vi "ROS_Service_Setup.vi"(4 "Msg to Send":string, 5 "Subscriber":T4, 6 "Log in":path, 7 "ROS":T1={"topic port"=1236, "Node"="/labview", "topic"="/robot/head/command_head_nod", "type"="std_msgs/Bool", "node port"=7000, "error "={"status"=FALSE, "code"=0, "source"=""}, "Direction"=enum."Publisher", "APIs"=[], "Update (ms)"=1, "write queue"=1}, 8 "Log in":T3[](array[typedef])) -> (0 "Log out":path, 1 "Success?":bool, 2 "Reply":string, 3 "Log out":T3[](array[typedef]))   [LabVIEW 2012]
doc: "Creates and sends the connection header and message to a service provider. Implemented in the background server."
uses:
  <userlib>/ROSforLV/ROS/Code/Console/Servers/ServerSubs/ROSLog.ctl
  <userlib>/ROSforLV/ROS/Code/SubVIs/_ROSControl.ctl
  <userlib>/ROSforLV/ROS/Code/SubVIs/_ROSDirection.ctl
  <userlib>/ROSforLV/ROS/Code/_ROSDefinition.vi
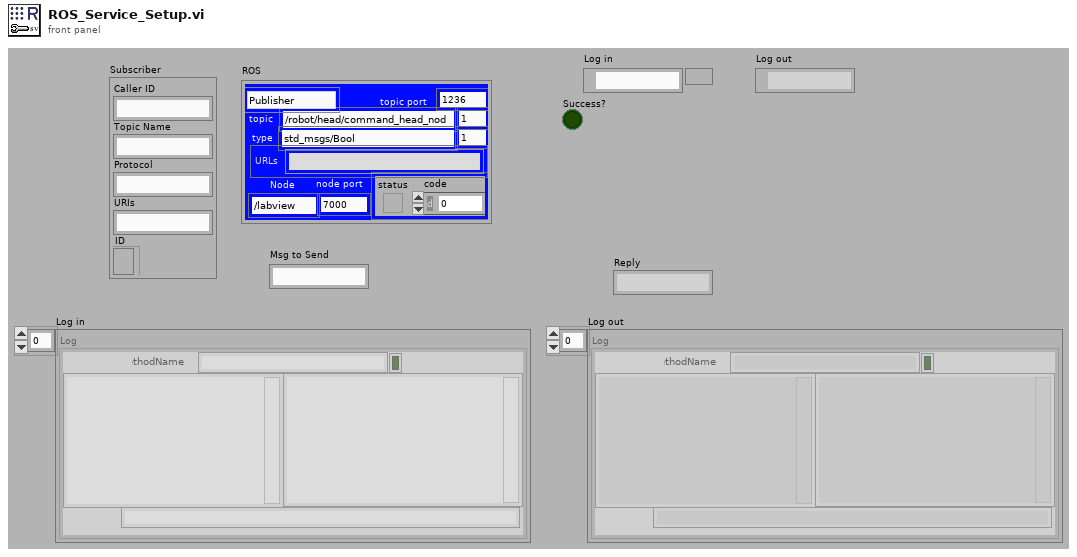
[diagram p1: front panel]
types:
  T1 = typedef "_ROSControl.ctl" = cluster{"topic port":u16, "Node":string, "topic":string, "type":string, "node port":u32, "error ":errorcluster, "Direction":T2, "APIs":string[], "Update (ms)":u16, "write queue":u16}
  T2 = typedef "_ROSDirection.ctl" = enum16{"Node", "Publisher", "Subscriber", "Service Client"}
  T3 = typedef "ROSLog.ctl" = cluster{"Sent":string, "Reply":string, "MethodName":string, "success":bool, "Dir1":string, "Dir2":string, "Time Stamp":string, "error":errorcluster, "Preamble":string}
  T4 = cluster{"Caller ID":string, "Topic Name":string, "Protocol":string, "URIs":string, "ID":refnum<k5>}
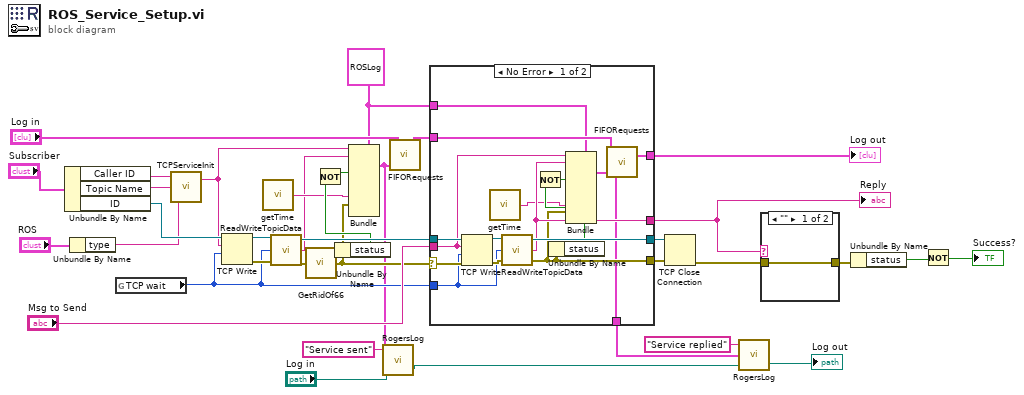
[diagram p0: block diagram]
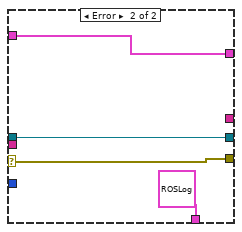
[diagram p2: hidden frame]
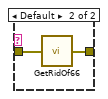
[diagram p3: hidden frame]
diagram:
  w16 = T3 {"Sent"="", "Reply"="", "MethodName"="Service", "success"=FALSE, "Dir1"="To ROS", "Dir2"="From ROS", "Time Stamp"="", "error"={"status"=FALSE, "code"=0, "source"=""}, "Preamble"=""} ("Log")
  n1 = Unbundle By Name("Subscriber") -> ("Caller ID"=w35:string, "Topic Name"=w34:string, "ID"=w28:refnum<k5>)
  n2 = Unbundle By Name("ROS") -> ("type"=w13:string)
  n3 = global read "_ROSDefinition.vi" "TCP wait"() -> (w12:i32)
  n4 = call <userlib>:"TCPServiceInit.vi"("Type"=w13, "topic"=w34, "callerID"=w35) -> ("TCP ROS Reply"=w24:string)  [unwired: 1 out]
  n5 = TCP Write(connection ID=w28, data in=w24, 9:w12) -> (connection ID out=w27:refnum<k5>, error out=w26:errorcluster)  [unwired: 1 in, 1 out]
  n6 = call <userlib>:"getTime.vi"() -> ("Current Time"=w17:string)  [unwired: 1 in]
  n7 = call <userlib>:"ReadWriteTopicData.vi"("error in (no error)"=w26, "timeout ms (1000)"=w12, "connection ID in"=w27) -> ("error out"=w18:errorcluster, "data out"=w15:string, "connection ID out"=w25:refnum<k5>)
  n8 = call <userlib>:"GetRidOf66.vi"("error in (no error)"=w18) -> ("error out"=w11:errorcluster)
  n9 = Unbundle By Name(w11) -> ("status"=w22:bool)
  n10 = Not(x=w22) -> (.not. x?=w21:bool)
  n11 = Bundle(cluster=w16, "Sent"=w24, "Reply"=w15, "success"=w21, "Time Stamp"=w17, "error"=w11) -> (w9:T3)  [unwired: 4 in]
  n12 = call <userlib>:"RogersLog.vi"("Text to add"="Service sent", "Log"=w9, "LogPath in"="Log in") -> ("LogPath out"=w7:path)  [unwired: 2 in, 1 out]
  n13 = call <userlib>:"FIFORequests.vi"("Log"=w9, "Requests in"="Log in") -> ("Requests out"=w19:T3[])  [unwired: 1 in]
  n14 = case shown="No Error" w11 {
    selector: w11 -> [w48 w55]
    tunnel: w25 -> [w50 w56]
    tunnel: w12 -> [w41 _]
    tunnel: [w49 w56] -> w23
    tunnel: [w38 w55] -> w20
    tunnel: w19 -> [w47 w54]
    tunnel: [w46 w54] -> w32
    tunnel: "Msg to Send" -> [w42 _]
    tunnel: [w43 _] -> w30
    tunnel: w16 -> [w39 _]
    tunnel: [w37 T3 {"Sent"="", "Reply"="", "MethodName"="No reply", "success"=FALSE, "Dir1"="", "Dir2"="", "Time Stamp"="", "error"={"status"=FALSE, "code"=0, "source"=""}, "Preamble"=""} ("Log")] -> w6
    frame No Error {
      n15 = TCP Write(connection ID=w50, data in=w42, error in (no error)=w48, 9:w41) -> (connection ID out=w52:refnum<k5>, error out=w51:errorcluster)  [unwired: 1 out]
      n16 = call <userlib>:"getTime.vi"() -> ("Current Time"=w40:string)  [unwired: 1 in]
      n17 = call <userlib>:"ReadWriteTopicData.vi"("error in (no error)"=w51, "timeout ms (1000)"=w41, "connection ID in"=w52) -> ("error out"=w38:errorcluster, "data out"=w43:string, "connection ID out"=w49:refnum<k5>)
      n18 = Unbundle By Name(w38) -> ("status"=w45:bool)
      n19 = Not(x=w45) -> (.not. x?=w44:bool)
      n20 = Bundle(cluster=w39, "Sent"=w42, "Reply"=w43, "success"=w44, "Time Stamp"=w40, "error"=w38) -> (w37:T3)  [unwired: 4 in]
      n21 = call <userlib>:"FIFORequests.vi"("Log"=w37, "Requests in"=w47) -> ("Requests out"=w46:T3[])  [unwired: 1 in]
    }
    frame Error {
    }
  }
  "Log out" <- w32
  "Reply" <- w30
  n22 = TCP Close Connection(connection ID=w23, error in (no error)=w20) -> (error out=w29:errorcluster)  [unwired: 1 in, 1 out]
  n23 = call <userlib>:"RogersLog.vi"("Text to add"="Service replied", "Log"=w6, "LogPath in"=w7) -> ("LogPath out"=→"Log out":path)  [unwired: 2 in, 1 out]
  n24 = case shown="\"\"" w30 {
    tunnel: w29 -> [w57 w59]
    tunnel: [w57 w58] -> w3
    frame "" {
    }
    frame Default {
      n25 = call <userlib>:"GetRidOf66.vi"("error in (no error)"=w59) -> ("error out"=w58:errorcluster)
    }
  }
  n26 = Unbundle By Name(w3) -> ("status"=w2:bool)
  n27 = Not(x=w2) -> (.not. x?=→"Success?":bool)
